vi "PID Output Rate Limiter (DBL Array).vi"(4 "reinitialize? (F)":bool, 6 "dt (s)":dbl=-1.0 format="%.2f", 7 "output rate (EGU/min)":dbl[](array[numeric])=[1.0] format="%.2f", 8 "initial output":dbl[](array[numeric])=[0.0] format="%.2f", 9 "input (controller output)":dbl[](array[numeric])=[0.0] format="%.2f") -> (0 "dt out (s)":dbl format="%.3f", 3 "output":dbl[](array[numeric]) format="%.2f")   [LabVIEW 2013]
doc: "This function can be used to specify a maximum rate of change of the controller output. Place this VI immediately after the PID VI in your control application."
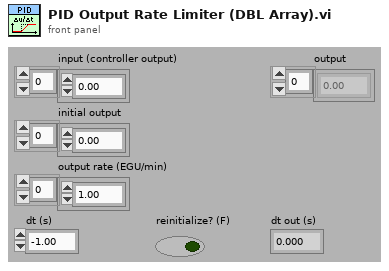
[diagram p1: front panel]
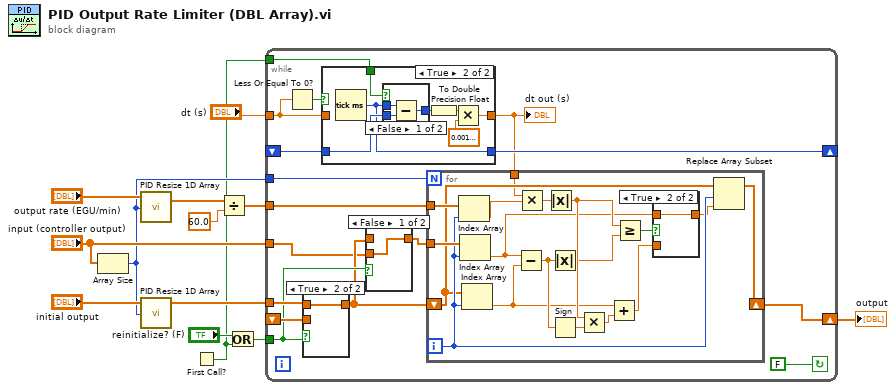
[diagram p0: block diagram]
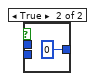
[diagram p4: hidden frame]
diagram:
  n1 = Array Size(array="input (controller output)") -> (size(s)=w4:i32)
  n2 = call "PID Resize 1D Array.vi"("array size"=w4, "input array"="output rate (EGU/min)") -> ("output array"=w6:dbl[])  [unwired: 3 in]
  n3 = call "PID Resize 1D Array.vi"("array size"=w4, "input array"="initial output") -> ("output array"=w8:dbl[])  [unwired: 3 in]
  n4 = First Call?() -> (First Call?: T/F=w1:bool)
  n5 = Divide(x=w6, y=60.0) -> (x/y=w5:dbl[])
  n6 = Or(x="reinitialize? (F)", y=w1) -> (x .or. y?=w12:bool)
  n7 = while {
    tunnel: w12 -> [w17]
    shift-left: _ -> [w21]
    shift-right: [w23] -> _
    shift-left: _ -> [w28]
    shift-right: [w24] -> w3
    tunnel: w5 -> [w26]
    tunnel: "input (controller output)" -> [w14]
    tunnel: w8 -> [w27]
    tunnel: w4 -> [w25]
    tunnel: "dt (s)" -> [w20]
    tunnel: w1 -> [w18]
    stop <- FALSE continue-if-true
    n8 = Less Or Equal To 0?(x=w20) -> (x <= 0?=w19:bool)
    n9 = case shown="True" w17 {
      tunnel: w28 -> [w45 _]
      tunnel: w27 -> [_ w46]
      tunnel: [w45 w46] -> w15
      frame False {
      }
      frame True {
      }
    }
    n10 = case shown="True" w19 {
      tunnel: [w33 w37] -> w22
      tunnel: w21 -> [w32 w36]
      tunnel: [w32 w35] -> w23
      tunnel: w20 -> [w33 _]
      tunnel: w18 -> [_ w34]
      frame False {
      }
      frame True {
        n11 = Tick Count (ms)() -> (millisecond timer value=w35:u32)
        n12 = case shown="False" w34 {
          tunnel: [w43 u32 0] -> w39
          tunnel: w36 -> [w42 _]
          tunnel: w35 -> [w41 _]
          frame False {
            n13 = Subtract(x=w41, y=w42) -> (x-y=w43:u32)
          }
          frame True {
          }
        }
        n14 = To Double Precision Float(number=w39) -> (double precision float=w38:dbl)
        n15 = Multiply(x=w38, y=0.0010000000474974513) -> (x*y=w37:dbl)
      }
    }
    "dt out (s)" <- w22
    n16 = case shown="False" w17 {
      tunnel: w14 -> [w30 _]
      tunnel: w15 -> [_ w31]
      tunnel: [w30 w31] -> w16
      frame False {
      }
      frame True {
      }
    }
    n17 = for {
      N: w25 -> [_]
      tunnel: w22 -> [w48]
      tunnel: w26 -> [w58]
      tunnel: w16 -> [w57]
      shift-right: [w53] -> w24
      shift-left: w15 -> [w54]
      i -> [w56]
      n18 = Index Array(array=w58, index=w56) -> (element=w47:dbl)
      n19 = Index Array(array=w57, index=w56) -> (element=w51:dbl)
      n20 = Index Array(array=w54, index=w56) -> (element=w55:dbl)
      n21 = Subtract(x=w51, y=w55) -> (x-y=w63:dbl)
      n22 = Multiply(x=w48, y=w47) -> (x*y=w64:dbl)
      n23 = Absolute Value(x=w64) -> (abs(x)=w61:dbl)
      n24 = Absolute Value(x=w63) -> (abs(x)=w59:dbl)
      n25 = Sign(1:w63) -> (0:w62:dbl)
      n26 = Multiply(x=w61, y=w62) -> (x*y=w60:dbl)
      n27 = Add(x=w55, y=w60) -> (x+y=w50:dbl)
      n28 = Greater Or Equal?(x=w61, y=w59) -> (x >= y?=w52:bool)
      n29 = case shown="True" w52 {
        tunnel: w51 -> [_ w66]
        tunnel: w50 -> [w65 _]
        tunnel: [w65 w66] -> w49
        frame False {
        }
        frame True {
        }
      }
      n30 = Replace Array Subset(array=w54, new element=w49, index=w56) -> (w53:dbl[])
    }
  }
  "output" <- w3
